vi "Do.vi"(8 "error in (no error)":errorcluster, 10 "Actor in":refnum<class "Actor.lvclass">, 11 "Meerstetter output":refnum<class "Meerstetter output.lvclass">) -> (0 "error out":errorcluster, 2 "Actor out":refnum<class "Actor.lvclass">)   [LabVIEW 2014, in "Meerstetter Lib.lvlib" / "Meerstetter output.lvclass"]
doc: "(<B>Filename</B>: Actor Framework.lvlib:Message.lvclass:Do.vi)\n\nDefines what a message does when it is received by an actor. Generally, a message instructs an actor to invoke one of its methods. By default, this method does nothing. A child class must override it to define behavior. Create a child class by using the Actor Framework Message Maker dialog box."
uses:
  Meerstetter output.lvclass
  <vilib>/ActorFramework/Actor/Actor.lvclass
  Meerstetter output.lvclass/Meerstetter output.ctl
  reusable/DAQ Device/Device/Device.lvclass
  Meerstetter TEC.lvclass
  reusable/DAQ Device/Device/Device.lvclass/Device.ctl
  SuperActor/SuperActor.lvclass/SuperActor.ctl
  reusable/DAQ Device/Device/Read Configurable Device.vi
  SuperActor/Read CVT Session.vi
  SuperActor/Read ID.vi
  <userlib>/_Session Fwk/Session - Root.lvclass
  Configurable Device/Configurable Device.lvclass
  reusable/Session APIs/CVT/CVT.lvclass
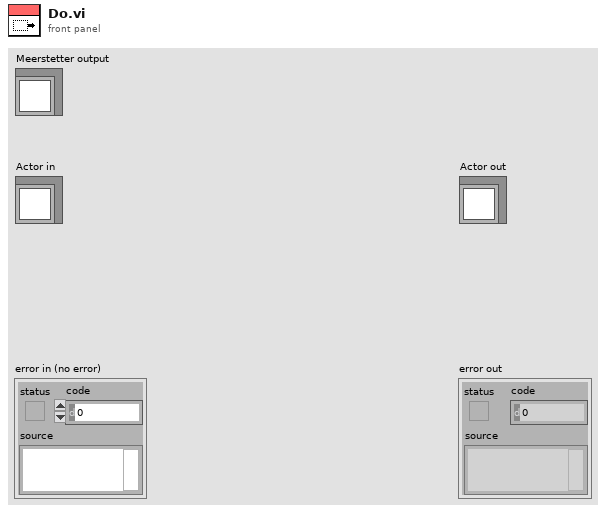
[diagram p1: front panel]
types:
  T1 = typedef "Session - Root.lvclass/Session Handle.ctl" = refnum<data-value>
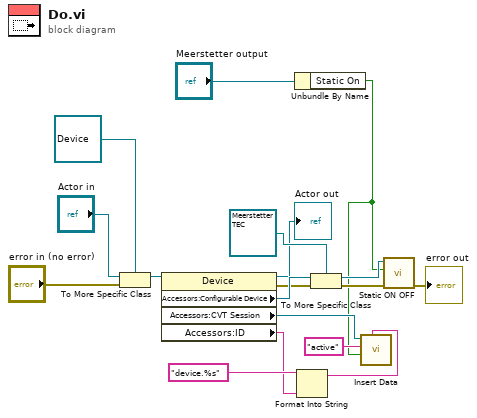
[diagram p0: block diagram]
diagram:
  n1 = To More Specific Class(target class=refnum<class "Device.lvclass"> refnum ("DAQ Device.lvlib:Device"), reference="Actor in", error in="error in (no error)") -> (specific class reference=w15:refnum<class "Device.lvclass">)  [unwired: 1 out]
  n2 = property class="Device"(reference=w15) -> (reference out=→"Actor out":refnum<class "Device.lvclass">, error out=w11:errorcluster, "Accessors:Configurable Device"=w12:refnum<class "Configurable Device.lvclass">, "Accessors:CVT Session"=w6:T1, "Accessors:ID"=w4:string)  [unwired: 1 in]
  n3 = Unbundle By Name("Meerstetter output") -> ("Static On"=w1:bool)
  n4 = Format Into String(format string="device.%s", w4) -> (resulting string=w3:string)  [unwired: 2 in, 1 out]
  n5 = To More Specific Class(target class=refnum<class "Meerstetter TEC.lvclass"> refnum ("Meerstetter Lib.lvlib:TEC 1090"), reference=w12, error in=w11) -> (specific class reference=w9:refnum<class "Meerstetter TEC.lvclass">, error out=w8:errorcluster)
  n6 = call "Insert Data.vi"("Group"=w3, "Data"=w1, "tag"="active", "CVT Session In"=w6) -> ()  [unwired: 6 in, 2 out]
  n7 = call "Static ON OFF.vi"("error in"=w8, "ON"=w1, "TEC 1090 in"=w9) -> ("error out"=→"error out":errorcluster)  [unwired: 7 in, 1 out]
